vi "ICS425 Read Write.vi"(8 "Error In":errorcluster, 10 "Cmd":string, 11 "VISA (Input)":refnum<visa-resource-name>) -> (0 "Error Out":errorcluster, 1 "concatenated input string":string, 2 "read buffer":string, 3 "VISA Refnum (Output)":refnum<visa-resource-name>)   [LabVIEW 2018]
panel:
  out "Serial Settings:Number of Bytes at Serial Port":u32
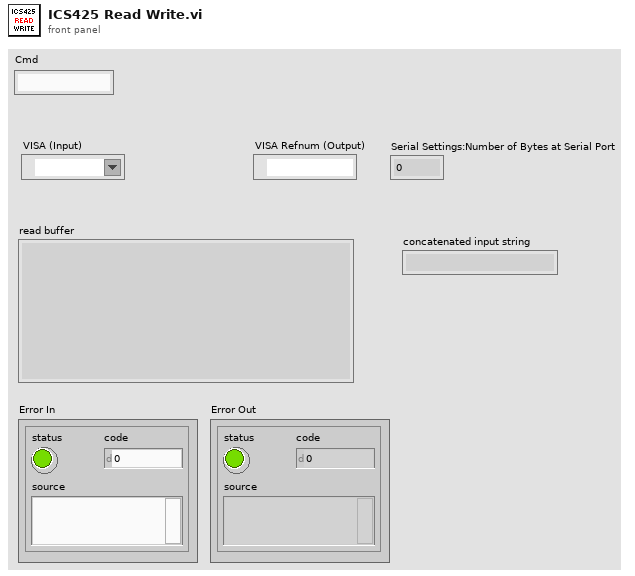
[diagram p1: front panel]
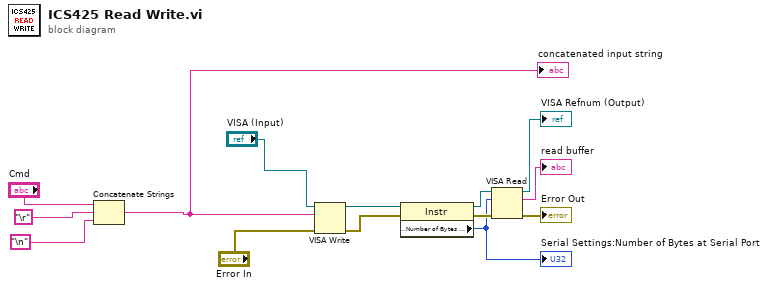
[diagram p0: block diagram]
diagram:
  n1 = Concatenate Strings("Cmd", "\r", "\n") -> (w1:string)
  "concatenated input string" <- w1
  n2 = VISA Write(VISA resource name="VISA (Input)", write buffer=w1, error in (no error)="Error In") -> (VISA resource name out=w5:refnum<visa-resource-name>, error out=w6:errorcluster)  [unwired: 1 out]
  n3 = property class="Instr"(reference=w5, error in=w6) -> (reference out=w12:refnum<visa-resource-name>, error out=w13:errorcluster, "Serial Settings:Number of Bytes at Serial Port"=w11:u32)
  "Serial Settings:Number of Bytes at Serial Port" <- w11
  n4 = VISA Read(VISA resource name=w12, byte count=w11, error in (no error)=w13) -> (VISA resource name out=→"VISA Refnum (Output)":refnum<visa-resource-name>, read buffer=→"read buffer":string, error out=→"Error Out":errorcluster)  [unwired: 1 out]
